vi "Station-SeqRun.vi"(8 "error in (no error)":errorcluster, 9 "BreakSource":T1, 10 "BreakReason":T3, 11 "State":T2) -> (0 "error out":errorcluster)   [LabVIEW 2016]
uses:
  Sequence/Sequence.Test.BreakReason.ctl
  Sequence/Sequence.State.ctl
  Sequence/Sequence.Test.BreakSource.ctl
  Station.Action.ctl
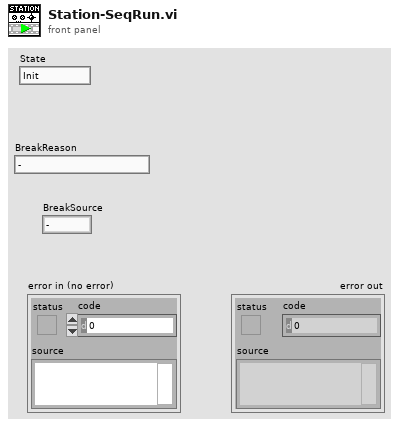
[diagram p1: front panel]
types:
  T1 = typedef "Sequence.Test.BreakSource.ctl" = enum16{"-", "A", "B", "A/B"}
  T2 = typedef "Sequence.State.ctl" = enum16{"Init", "Idle", "Home", "Work", "Run", "Pause"}
  T3 = typedef "Sequence.Test.BreakReason.ctl" = enum16{"-", "NOK container", "OK container", "Rev empty", "Rev missing", "Rev wrong", "Fork missing", "Fork wrong", "NOK limit", "Unload failure", "Single slot", "Part done", "Err: Prod move work", "Err: Prod move home", "Err: Prod lift work", "Err: Prod lift home", "Err: Prod Arm Work", "Err: Prod Arm NOK", "Err: Prod Arm OK", "Err: Prod NOK suck", "Err: Prod NOK drop", "Err: Prod OK missing", "Err: Prod OK suck", "Err: Prod OK drop"}
  T4 = cluster{"State":T2, "BreakReason":T3, "BreakSource":T1}
  T5 = typedef "Station.Action.ctl" = enum32{"idle", "constructor", "destructor", "--- Station ---", "Hardware.Init", "Status.Update", "Status.Clear", "Order", "Init", "Ready", "Start", "Run", "Stop", "Error", "Home", "Done", "Seq.Run", "Seq.Done", "Tower.Update", "Mode.Select", "Emg", "Emg.Reset", "Emg.Check", "Home.Check", "Prod.Check", "Butt.Check"}
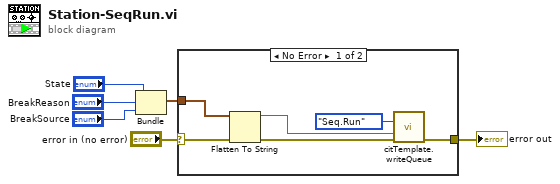
[diagram p0: block diagram]
diagram:
  n1 = Bundle("State"="State", "BreakReason"="BreakReason", "BreakSource"="BreakSource") -> (w3:T4)  [unwired: 1 in]
  n2 = case shown="No Error" "error in (no error)" {
    selector: "error in (no error)" -> [w10 w13]
    tunnel: [w12 w13] -> w6
    tunnel: w3 -> [w7 _]
    frame No Error {
      n3 = Flatten To String(anything=w7, error in (no error)=w10) -> (data string=w8:string, error out=w9:errorcluster)  [unwired: 2 in, 1 out]
      n4 = call "citTemplate.writeQueue.vi"("event in (if not connected:all statemachine with data event)"=Station.Action."Seq.Run" ("Action"), "data in"=w8, "error in (no error)"=w9) -> ("error out"=w12:errorcluster)  [unwired: 12 in]
    }
    frame Error {
    }
  }
  "error out" <- w6
